vi "Safety Config Motor.vi"() -> ()   [LabVIEW 2025]
doc: "This example shows how to set up Safety Config for a motor. The Safety Config VI is called after Motor Open. It is set to enable with a timeout of 0.1 seconds (100 ms). This means the motor control loop must run at least this fast to keep the Safety Config from pausing the motor.\n\n1. Set up your motor and wiring.\n2. Run this VI.\n3. Increase the Speed until a motor is running.\n4. Increase the loop delay to 300 ms. This simulates what happens if other code is starving the motor loop code. When the loop delay is large enough, the Safety Config will turn off the motor. You will likely see the motor pulse on and off, because when Safety Config is enabled Motor Set Output needs to be called at least every 100 ms.\n\nThis VI shows how to enable Safety Config. See other Safety Config examples to see how to turn Safety Config on and off while your program is running.\n\nThis example expects a USB cable connected from your development PC to the Type B USB Jack (next to the power input) on the roboRIO.\n\nThis example requires the Driver Station to be running with Teleoperated Enabled."
uses:
  <vilib>/Rock Robotics/SystemInterfaces/DIO/FPGA_DIOPWMChannel.ctl
  <vilib>/Rock Robotics/WPI/SafetyOutput/WPI_SafetyOutputConfigMenu.ctl
  <vilib>/Rock Robotics/WPI/MotorControl/WPI_MotorControlOpen Talon.vi
panel:
  in  "loop delay (ms)":u32(slide)=20 scale=0.0..300.0
  in  "Speed (-1 to 1)":dbl(slide) min=-1.0 max=1.0 step=0.1 scale=-1.0..1.0 scale format="%#.3f"
  in  "PWM Channel":T1
  in  "stop":bool
  # "Set this input before running."
  # "This can be set while running."
  # "This example requires the Driver Station to be running with Teleoperated Enabled."
  # "PWM cable"
  # "This shows wiring for a Talon speed controller.  The wiring is similar for other motor controllers.  If you change the controller type, you must also select the appropriate instance of the Motor Open VI on the diagram."
  # "Power\nTerminals"
  # "Motor\nTerminals"
  # "+"
  # "+"
  # "M"
  # "B"
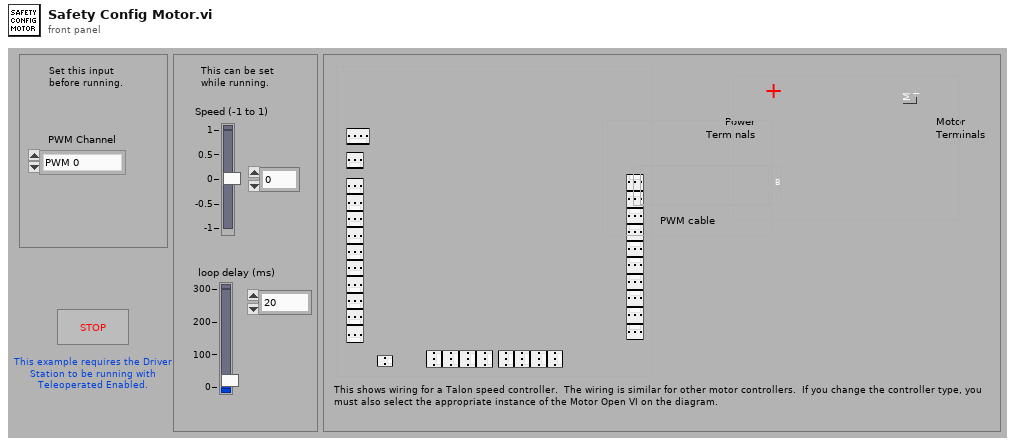
[diagram p1: front panel]
types:
  T1 = typedef "FPGA_DIOPWMChannel.ctl" = enum8{"PWM 0", "PWM 1", "PWM 2", "PWM 3", "PWM 4", "PWM 5", "PWM 6", "PWM 7", "PWM 8", "PWM 9", "PWM MXP 0", "PWM MXP 1", "PWM MXP 2", "PWM MXP 3", "PWM MXP 4", "PWM MXP 5", "PWM MXP 6", "PWM MXP 7", "PWM MXP 8", "PWM MXP 9", "Invalid"}
  T2 = typedef "WPI_SafetyOutputConfigMenu.ctl" = enum16{"Enable", "Disable"}
  T3 = typedef "WPI_MotorControlDeviceRef.ctl" = cluster{"DeviceStatus":errorcluster, "Type":T4, "PWM":cluster{"PWM Channel":T1, "DeadBand":T5}, "CAN":cluster{"Device Number":u8, "SetOutput VI Ref":variant, "GetOutput VI Ref":variant, "Enable VI Ref":variant, "Disable VI Ref":variant, "Data":variant}, "Invert":bool, "DIO PWM":cluster{"PWM \"Enable\" Channel":T1, "DIOChannel":T6, "PWM Rate":dbl}}
  T4 = typedef "WPI_MotorControlType.ctl" = enum16{"PWM", "CAN", "DIO PWM"}
  T5 = typedef "WPI_PWMDeadband.ctl" = cluster{"Name":string, "maxPositivePwm":i32, "minPositivePwm":i32, "centerPwm":i32, "maxNegativePwm":i32, "minNegativePwm":i32, "angularRange":u16}
  T6 = typedef "FPGA_DIOChannel.ctl" = enum8{"DIO 0", "DIO 1", "DIO 2", "DIO 3", "DIO 4", "DIO 5", "DIO 6", "DIO 7", "DIO 8", "DIO 9", "DIO MXP 0", "DIO MXP 1", "DIO MXP 2", "DIO MXP 3", "DIO MXP 4", "DIO MXP 5", "DIO MXP 6", "DIO MXP 7", "DIO MXP 8", "DIO MXP 9", "DIO MXP 10", "DIO MXP 11", "DIO MXP 12", "DIO MXP 13", "DIO MXP 14", "DIO MXP 15", "SPI Port CS1", "SPI Port CS2", "SPI Port CS3", "SPI Port MISO", "SPI Port MOSI", "Invalid"}
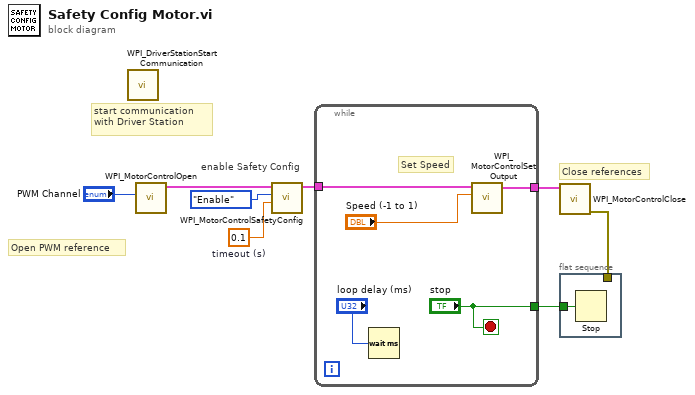
[diagram p0: block diagram]
diagram:
  w3 = 0.1  # timeout (s)
  # "enable Safety Config"
  # "start communication with Driver Station"
  # "Close references"
  # "Open PWM reference"
  n1 = call <vilib>:"WPI_DriverStationStart Communication.vi"() -> ()  [unwired: 3 in, 9 out]
  n2 = call-poly <vilib>:"WPI_MotorControlOpen.vi"("PWM Channel"="PWM Channel") -> ("MotorControlDeviceRef"=w6:T3)  [unwired: 3 in, 7 out]
  n3 = call <vilib>:"WPI_MotorControlSafetyConfig.vi"("timeout (s)"=w3, "mode"=WPI_SafetyOutputConfigMenu."Enable", "MotorControlDevRef"=w6) -> ("MotorControlDevRef"=w5:T3)  [unwired: 1 in, 7 out]
  n4 = while {
    tunnel: w5 -> [w13]
    tunnel: [w11] -> w7
    tunnel: ["stop"] -> w2
    stop <- "stop" stop-if-true
    # "Set Speed"
    n5 = Wait (ms)(milliseconds to wait="loop delay (ms)") -> ()  [unwired: 1 out]
    n6 = call <vilib>:"WPI_MotorControlSetOutput.vi"("Output"="Speed (-1 to 1)", "MotorControlDevRef"=w13) -> ("MotorControlDevRef"=w11:T3)  [unwired: 2 in, 7 out]
  }
  n7 = call <vilib>:"WPI_MotorControlClose.vi"("MotorControlDevRef"=w7) -> ("error out"=w1:errorcluster)  [unwired: 1 in, 9 out]
  n8 = flat-sequence {
    tunnel: w2 -> [w14]
    tunnel: w1 -> [_]
    frame #0 {
      n9 = Stop(stop? (T)=w14) -> ()
    }
  }
